vi "Match Multiplexer.vi"(8 "error in":errorcluster, 10 "Frame Data":u8[](array[numeric]), 11 "SDO Transfer in":refnum<class "SDO Transfer.lvclass">) -> (0 "error out":errorcluster, 2 "Match":bool, 3 "SDO Transfer out":refnum<class "SDO Transfer.lvclass">)   [LabVIEW 2020, in "CANopen.lvlib" / "SDO Manager.lvlib" / "SDO Transfer.lvclass"]
uses:
  SDO Transfer.lvclass
  SDO Transfer.lvclass/SDO Transfer.ctl
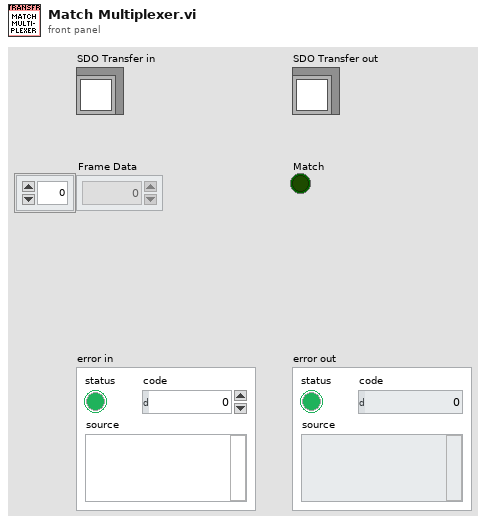
[diagram p1: front panel]
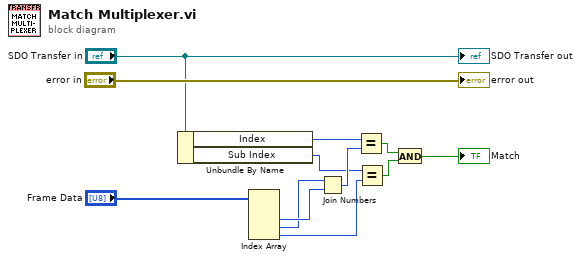
[diagram p0: block diagram]
diagram:
  n1 = Unbundle By Name("SDO Transfer in") -> ("Index"=w2:u16, "Sub Index"=w1:u8)
  n2 = Index Array(array="Frame Data") -> (element #2=w12:u8, element #3=w11:u8, element #4=w10:u8)  [unwired: 4 in, 1 out]
  n3 = Join Numbers(hi=w11, lo=w12) -> ((hi.lo)=w6:u16)
  n4 = Equal?(x=w2, y=w6) -> (x = y?=w8:bool)
  n5 = Equal?(x=w1, y=w10) -> (x = y?=w9:bool)
  n6 = And(x=w8, y=w9) -> (x .and. y?=→"Match":bool)
  "SDO Transfer out" <- "SDO Transfer in"
  "error out" <- "error in"
